vi "fpga_W&R_ADCs_W_3DAC.vi"() -> ()   [LabVIEW 2018]
uses:
  <vilib>/rvi/Emulation/niFpgaGetClockAttributes.vi
  <vilib>/rvi/Emulation/niFpgaSctlEmulationGetInTimedLoop.vi
  <vilib>/rvi/Emulation/niFpgaEmulationReportErrorSimple.vi
  <vilib>/rvi/eio/common/nirviEmuTemplateMethod_errors.vi
  <vilib>/rvi/Emulation/niFpgaCriticalErrorInLSC.vi
  <vilib>/eio/EIONode/EIONode.xnode
panel:
  in  "DAC 3 write":bool[](array[boolean])=[FALSE, TRUE, TRUE, TRUE, TRUE, TRUE, TRUE, TRUE, TRUE, TRUE, TRUE, TRUE, TRUE, TRUE, TRUE, TRUE]
  in  "DAC 2 write":bool[](array[boolean])=[FALSE, TRUE, TRUE, TRUE, TRUE, TRUE, TRUE, TRUE, TRUE, TRUE, TRUE, TRUE, TRUE, TRUE, TRUE, TRUE]
  in  "DAC 1 write":bool[](array[boolean])=[FALSE, TRUE, TRUE, TRUE, TRUE, TRUE, TRUE, TRUE, TRUE, TRUE, TRUE, TRUE, TRUE, TRUE, TRUE, TRUE]
  out "ADC read":bool[](array[boolean])=[FALSE, FALSE, FALSE, TRUE, TRUE, TRUE, FALSE, TRUE, FALSE, TRUE, FALSE, FALSE, FALSE, TRUE, FALSE, FALSE]
  in  "ADC write":bool[](array[boolean])=[FALSE, FALSE, FALSE, FALSE, FALSE, TRUE, FALSE, FALSE, FALSE, FALSE, FALSE, FALSE, FALSE, FALSE, FALSE, FALSE]
  in  "delay (us)":u32=40000
  in  "Stop":bool
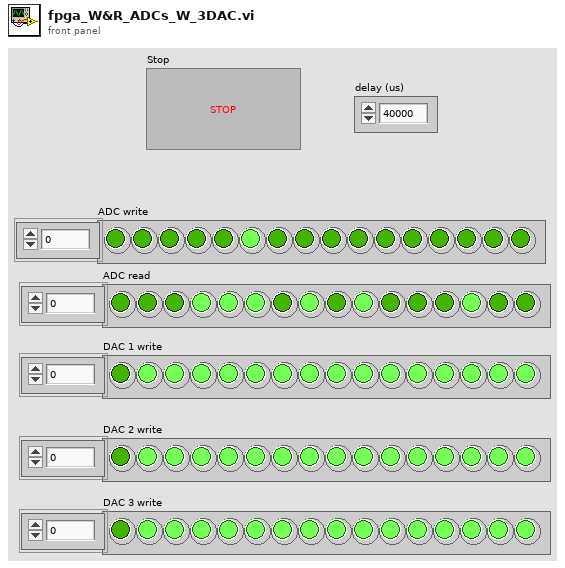
[diagram p1: front panel]
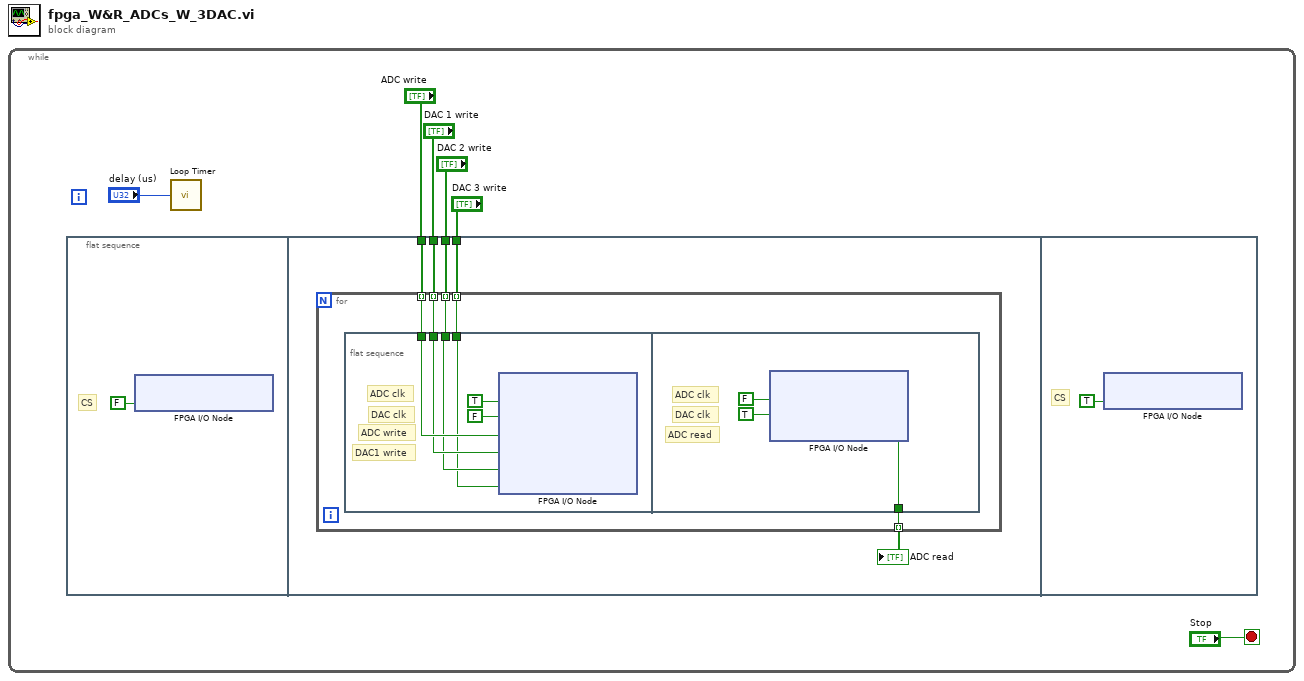
[diagram p0: block diagram]
diagram:
  n1 = while {
    stop <- "Stop" stop-if-true
    n2 = flat-sequence {
      tunnel: "DAC 1 write" -> [w12]
      tunnel: "ADC write" -> [w11]
      tunnel: "DAC 2 write" -> [w9]
      tunnel: "DAC 3 write" -> [w8]
      frame #0 {
        # "CS"
        n3 = xnode "FPGA I/O Node"("ConnectorA/DIO4"=FALSE) -> ()  [unwired: 1 in, 1 out]
      }
      frame #1 {
        n4 = for {
          tunnel: w12 -> [w17] mode=indexing
          tunnel: w11 -> [w16] mode=indexing
          tunnel: [w15] -> w10 mode=indexing
          tunnel: w9 -> [w14] mode=indexing
          tunnel: w8 -> [w13] mode=indexing
          n5 = flat-sequence {
            tunnel: w17 -> [w20]
            tunnel: w16 -> [w21]
            tunnel: w14 -> [w19]
            tunnel: w13 -> [w18]
            tunnel: [w24] -> w15
            frame #0 {
              # "DAC1 write"
              # "ADC write"
              # "DAC clk"
              # "ADC clk"
              n6 = xnode "FPGA I/O Node"("ConnectorA/DIO3"=TRUE, "ConnectorA/DIO5"=FALSE, "ConnectorA/DIO2"=w21, "ConnectorA/DIO6"=w20, "ConnectorA/DIO7"=w19, "ConnectorA/DIO8"=w18) -> ()  [unwired: 6 in, 6 out]
            }
            frame #1 {
              # "ADC read"
              # "DAC clk"
              # "ADC clk"
              n7 = xnode "FPGA I/O Node"("ConnectorA/DIO3"=FALSE, "ConnectorA/DIO5"=TRUE) -> ("ConnectorA/DIO1"=w24:bool)  [unwired: 3 in, 3 out]
            }
          }
        }
        "ADC read" <- w10
      }
      frame #2 {
        # "CS"
        n8 = xnode "FPGA I/O Node"("ConnectorA/DIO4"=TRUE) -> ()  [unwired: 1 in, 1 out]
      }
    }
    n9 = call "Loop Timer"("Count(Ticks)"="delay (us)") -> ()  [unwired: 1 out]
  }
